vi "Read Name.vi"(11 "RelayInterface in":refnum<class "RelayInterface.lvclass">) -> (2 "Name":string, 3 "RelayInterface out":refnum<class "RelayInterface.lvclass">)   [LabVIEW 2015, in "SLSC Switch.lvlib" / "RelayInterface.lvclass"]
doc: "This reads the name of the relay"
uses:
  RelayInterface.lvclass
  RelayInterface.lvclass/RelayInterface.ctl
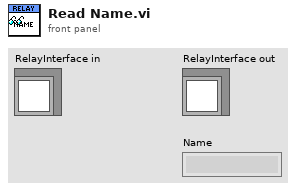
[diagram p1: front panel]
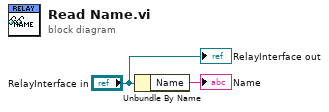
[diagram p0: block diagram]
diagram:
  n1 = Unbundle By Name("RelayInterface in") -> ("Name"=→"Name":string)
  "RelayInterface out" <- "RelayInterface in"
